vi "短信告警.vi"   [LabVIEW 2016]
uses:
  API/RND/example/Process var.vi
types:
  T1 = cluster{"水样参数输出":cluster{"mean":dbl, "变异系数":dbl, "随机数？":bool}, "零点参数输出":cluster{"mean":dbl, "变异系数":dbl, "随机数？":bool}, "跨度参数输出":cluster{"mean":dbl, "变异系数":dbl, "随机数？":bool}}
  T2 = cluster{"系统时间":timestamp, "工作状态":enum16{"空闲", "水样测试", "标样核查", "零点核查", "跨度核查", "空白测试", "平行样测试", "加标回收", "空白校准", "标样校准", "初始化（清洗）"}, "测量模式":enum16{"待机", "连续模式", "周期模式", "定点模式", "受控模式", "手动模式"}, "告警代码":u16, "故障代码":u16, "日志代码":u16, "软件版本":u16, "F0":sgl, "F1":sgl, "F2":sgl, "F3":sgl, "T":sgl, "H":sgl, "id":u16, "flowid":u16, "量程":u16, "总磷控温温度1":sgl, "营养盐控温温度2":sgl, "ADC":sgl}
  T3 = enum16{"空闲", "水样测试", "标样核查", "零点核查", "跨度核查", "空白测试", "平行样测试", "加标回收", "空白校准", "标样校准", "初始化（清洗）"}
  T4 = cluster{"参数":string, "报警内容":string, "报警分析":string}
  T5 = cluster{"系统时间":timestamp, "工作状态":u16, "测量模式":u16, "告警代码":u16, "故障代码":u16, "日志代码":u16, "软件版本":u16, "F0":sgl, "F1":sgl, "F2":sgl, "F3":sgl, "T":sgl, "H":sgl, "id":u16, "flowid":u16, "量程":u16}
  T6 = cluster{"ORP故障":bool, "温控器故障":bool, "加热故障":bool, "高锰酸钾报警":bool, "草酸钠报警":bool, "测量错误":bool, "校零错误":bool, "校标错误":bool, " 进水样超量程":bool, "排液阀故障":bool, "60分钟超时报警":bool, "进样无液体报警":bool}
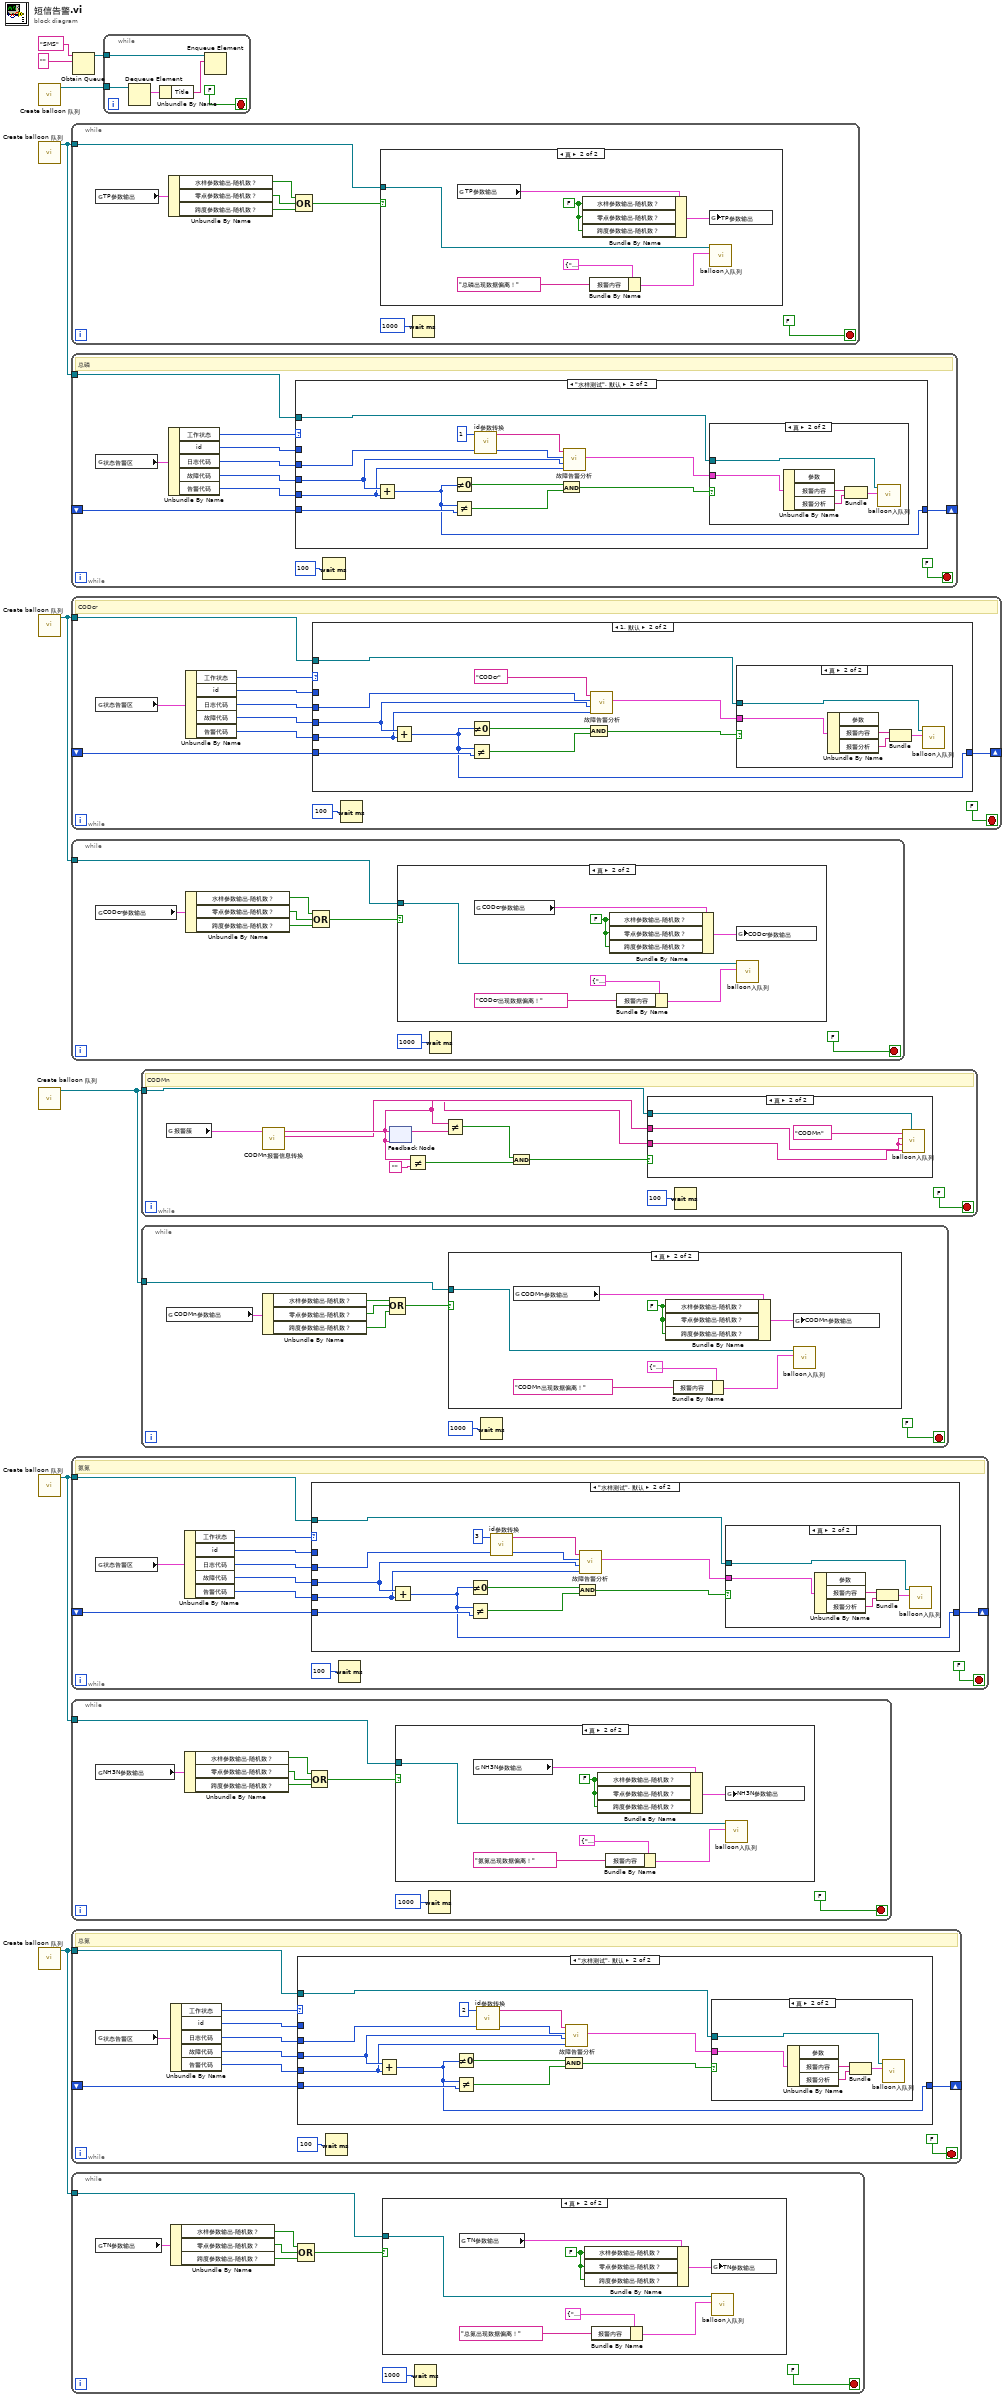
[diagram p0: block diagram]
diagram:
  n1 = call "Create balloon 队列.vi"() -> ("队列输出"=w9:refnum<queue>)  [unwired: 11 in]
  n2 = call "Create balloon 队列.vi"() -> ("队列输出"=w5:refnum<queue>)  [unwired: 11 in]
  n3 = call "Create balloon 队列.vi"() -> ("队列输出"=w4:refnum<queue>)  [unwired: 11 in]
  n4 = call "Create balloon 队列.vi"() -> ("队列输出"=w3:refnum<queue>)  [unwired: 11 in]
  n5 = call "Create balloon 队列.vi"() -> ("队列输出"=w2:refnum<queue>)  [unwired: 11 in]
  n6 = call "Create balloon 队列.vi"() -> ("队列输出"=w1:refnum<queue>)  [unwired: 11 in]
  n7 = while {
    tunnel: w5 -> [w10]
    stop <- FALSE stop-if-true
    n8 = global read "Process var.vi" "TP参数输出"() -> (w16:T1)
    n9 = Unbundle By Name(w16) -> ("水样参数输出.随机数？"=w15:bool, "零点参数输出.随机数？"=w14:bool, "跨度参数输出.随机数？"=w13:bool)
    n10 = Compound Arithmetic op=OR ("复合运算")(w15, w14, w13) -> (w12:bool)
    n11 = case shown="真" w12 {
      tunnel: w10 -> [_ w21]
      frame False {
      }
      frame True {
        w24 = FALSE ("水样参数输出.随机数？")
        n12 = global read "Process var.vi" "TP参数输出"() -> (w22:T1)
        n13 = Bundle By Name(cluster=w22, "水样参数输出.随机数？"=w24, "零点参数输出.随机数？"=w24, "跨度参数输出.随机数？"=w24) -> (w23:T1)
        n14 = Bundle By Name(cluster=cluster{"报警内容":string, "报警分析":string} {"报警内容"="", "报警分析"=""} ("报警内容"), "报警内容"="总磷出现数据偏离！") -> (w19:cluster{"报警内容":string, "报警分析":string})
        n15 = global write "Process var.vi" "TP参数输出"(w23) -> ()
        n16 = call "balloon入队列.vi"("报警内容"=w19, "队列"=w21) -> ()  [unwired: 9 in, 1 out]
      }
    }
    n17 = Wait (ms)(milliseconds to wait=u32 1000 ("等待时间（毫秒）")) -> ()  [unwired: 1 out]
  }
  n18 = while {
    tunnel: w5 -> [w31]
    shift-right: [w27] -> _
    shift-left: _ -> [w28]
    stop <- FALSE stop-if-true
    # "总磷"
    n19 = global read "VAR总磷总氮全局变量.vi" "状态告警区"() -> (w25:T2)
    n20 = Unbundle By Name(w25) -> ("工作状态"=w26:T3, "id"=w33:u16, "日志代码"=w32:u16, "故障代码"=w30:u16, "告警代码"=w29:u16)
    n21 = case shown="\"水样测试\", 默认" w26 {
      tunnel: w33 -> [_ _]
      tunnel: w32 -> [_ w48]
      tunnel: w31 -> [_ w45]
      tunnel: w30 -> [_ w44]
      tunnel: w29 -> [_ w43]
      tunnel: w28 -> [w36 w42]
      tunnel: [w36 w41] -> w27
      frame "空闲" {
      }
      frame "水样测试", Default {
        n22 = Add(x=w44, y=w43) -> (x+y=w41:u16)
        n23 = Not Equal To 0?(x=w41) -> (x != 0?=w40:bool)
        n24 = Not Equal?(x=w41, y=w42) -> (x != y?=w39:bool)
        n25 = call "id参数转换.vi"("id"=u16 1) -> ("table输出"=w46:string)  [unwired: 10 in]
        n26 = And(x=w40, y=w39) -> (x .and. y?=w38:bool)
        n27 = call "故障告警分析.vi"("告警代码"=w43, "故障代码"=w44, "运行步序"=w48, "参数"=w46) -> ("报警内容"=w47:T4)  [unwired: 6 in, 1 out]
        n28 = case shown="真" w38 {
          tunnel: w47 -> [_ w53]
          tunnel: w45 -> [_ w52]
          frame False {
          }
          frame True {
            n29 = Unbundle By Name(w53) -> ("报警内容"=w51:string, "报警分析"=w50:string)  [unwired: 1 out]
            n30 = Bundle("报警内容"=w51, "报警分析"=w50) -> (w49:cluster{"报警内容":string, "报警分析":string})  [unwired: 1 in]
            n31 = call "balloon入队列.vi"("报警内容"=w49, "队列"=w52) -> ()  [unwired: 9 in, 1 out]
          }
        }
      }
    }
    n32 = Wait (ms)(milliseconds to wait=u32 100) -> ()  [unwired: 1 out]
  }
  n33 = while {
    tunnel: w4 -> [w60]
    shift-right: [w56] -> _
    shift-left: _ -> [w57]
    stop <- FALSE stop-if-true
    # "CODcr"
    n34 = global read "CODcr全局变量.vi" "状态告警区"() -> (w54:T5)
    n35 = Unbundle By Name(w54) -> ("工作状态"=w55:u16, "id"=w62:u16, "日志代码"=w61:u16, "故障代码"=w59:u16, "告警代码"=w58:u16)
    n36 = case shown="1, 默认" w55 {
      tunnel: w62 -> [_ _]
      tunnel: w61 -> [_ w76]
      tunnel: w60 -> [_ w74]
      tunnel: w59 -> [_ w73]
      tunnel: w58 -> [_ w72]
      tunnel: w57 -> [w65 w71]
      tunnel: [w65 w70] -> w56
      frame 0 {
      }
      frame 1, Default {
        n37 = Add(x=w73, y=w72) -> (x+y=w70:u16)
        n38 = Not Equal To 0?(x=w70) -> (x != 0?=w69:bool)
        n39 = Not Equal?(x=w70, y=w71) -> (x != y?=w68:bool)
        n40 = And(x=w69, y=w68) -> (x .and. y?=w67:bool)
        n41 = call "故障告警分析.vi"("告警代码"=w72, "故障代码"=w73, "运行步序"=w76, "参数"="CODcr") -> ("报警内容"=w75:T4)  [unwired: 6 in, 1 out]
        n42 = case shown="真" w67 {
          tunnel: w75 -> [_ w81]
          tunnel: w74 -> [_ w80]
          frame False {
          }
          frame True {
            n43 = Unbundle By Name(w81) -> ("报警内容"=w79:string, "报警分析"=w78:string)  [unwired: 1 out]
            n44 = Bundle("报警内容"=w79, "报警分析"=w78) -> (w77:cluster{"报警内容":string, "报警分析":string})  [unwired: 1 in]
            n45 = call "balloon入队列.vi"("报警内容"=w77, "队列"=w80) -> ()  [unwired: 9 in, 1 out]
          }
        }
      }
    }
    n46 = Wait (ms)(milliseconds to wait=u32 100) -> ()  [unwired: 1 out]
  }
  n47 = while {
    tunnel: w4 -> [w82]
    stop <- FALSE stop-if-true
    n48 = global read "Process var.vi" "CODcr参数输出"() -> (w88:T1)
    n49 = Unbundle By Name(w88) -> ("水样参数输出.随机数？"=w87:bool, "零点参数输出.随机数？"=w86:bool, "跨度参数输出.随机数？"=w85:bool)
    n50 = Compound Arithmetic op=OR ("复合运算")(w87, w86, w85) -> (w84:bool)
    n51 = case shown="真" w84 {
      tunnel: w82 -> [_ w93]
      frame False {
      }
      frame True {
        w96 = FALSE ("水样参数输出.随机数？")
        n52 = global read "Process var.vi" "CODcr参数输出"() -> (w94:T1)
        n53 = Bundle By Name(cluster=w94, "水样参数输出.随机数？"=w96, "零点参数输出.随机数？"=w96, "跨度参数输出.随机数？"=w96) -> (w95:T1)
        n54 = Bundle By Name(cluster=cluster{"报警内容":string, "报警分析":string} {"报警内容"="", "报警分析"=""} ("报警内容"), "报警内容"="CODcr出现数据偏离！") -> (w91:cluster{"报警内容":string, "报警分析":string})
        n55 = global write "Process var.vi" "CODcr参数输出"(w95) -> ()
        n56 = call "balloon入队列.vi"("报警内容"=w91, "队列"=w93) -> ()  [unwired: 9 in, 1 out]
      }
    }
    n57 = Wait (ms)(milliseconds to wait=u32 1000 ("等待时间（毫秒）")) -> ()  [unwired: 1 out]
  }
  n58 = while {
    tunnel: w2 -> [w103]
    shift-right: [w99] -> _
    shift-left: _ -> [w100]
    stop <- FALSE stop-if-true
    # "氨氮"
    n59 = global read "VAR氨氮全局变量.vi" "状态告警区"() -> (w97:T2)
    n60 = Unbundle By Name(w97) -> ("工作状态"=w98:T3, "id"=w105:u16, "日志代码"=w104:u16, "故障代码"=w102:u16, "告警代码"=w101:u16)
    n61 = case shown="\"水样测试\", 默认" w98 {
      tunnel: w105 -> [_ _]
      tunnel: w104 -> [_ w120]
      tunnel: w103 -> [_ w117]
      tunnel: w102 -> [_ w116]
      tunnel: w101 -> [_ w115]
      tunnel: w100 -> [w108 w114]
      tunnel: [w108 w113] -> w99
      frame "空闲" {
      }
      frame "水样测试", Default {
        n62 = Add(x=w116, y=w115) -> (x+y=w113:u16)
        n63 = Not Equal To 0?(x=w113) -> (x != 0?=w112:bool)
        n64 = Not Equal?(x=w113, y=w114) -> (x != y?=w111:bool)
        n65 = call "id参数转换.vi"("id"=u16 3) -> ("table输出"=w118:string)  [unwired: 10 in]
        n66 = And(x=w112, y=w111) -> (x .and. y?=w110:bool)
        n67 = call "故障告警分析.vi"("告警代码"=w115, "故障代码"=w116, "运行步序"=w120, "参数"=w118) -> ("报警内容"=w119:T4)  [unwired: 6 in, 1 out]
        n68 = case shown="真" w110 {
          tunnel: w119 -> [_ w125]
          tunnel: w117 -> [_ w124]
          frame False {
          }
          frame True {
            n69 = Unbundle By Name(w125) -> ("报警内容"=w123:string, "报警分析"=w122:string)  [unwired: 1 out]
            n70 = Bundle("报警内容"=w123, "报警分析"=w122) -> (w121:cluster{"报警内容":string, "报警分析":string})  [unwired: 1 in]
            n71 = call "balloon入队列.vi"("报警内容"=w121, "队列"=w124) -> ()  [unwired: 9 in, 1 out]
          }
        }
      }
    }
    n72 = Wait (ms)(milliseconds to wait=u32 100) -> ()  [unwired: 1 out]
  }
  n73 = while {
    tunnel: w2 -> [w126]
    stop <- FALSE stop-if-true
    n74 = global read "Process var.vi" "NH3N参数输出"() -> (w132:T1)
    n75 = Unbundle By Name(w132) -> ("水样参数输出.随机数？"=w131:bool, "零点参数输出.随机数？"=w130:bool, "跨度参数输出.随机数？"=w129:bool)
    n76 = Compound Arithmetic op=OR ("复合运算")(w131, w130, w129) -> (w128:bool)
    n77 = case shown="真" w128 {
      tunnel: w126 -> [_ w137]
      frame False {
      }
      frame True {
        w140 = FALSE ("水样参数输出.随机数？")
        n78 = global read "Process var.vi" "NH3N参数输出"() -> (w138:T1)
        n79 = Bundle By Name(cluster=w138, "水样参数输出.随机数？"=w140, "零点参数输出.随机数？"=w140, "跨度参数输出.随机数？"=w140) -> (w139:T1)
        n80 = Bundle By Name(cluster=cluster{"报警内容":string, "报警分析":string} {"报警内容"="", "报警分析"=""} ("报警内容"), "报警内容"="氨氮出现数据偏离！") -> (w135:cluster{"报警内容":string, "报警分析":string})
        n81 = global write "Process var.vi" "NH3N参数输出"(w139) -> ()
        n82 = call "balloon入队列.vi"("报警内容"=w135, "队列"=w137) -> ()  [unwired: 9 in, 1 out]
      }
    }
    n83 = Wait (ms)(milliseconds to wait=u32 1000 ("等待时间（毫秒）")) -> ()  [unwired: 1 out]
  }
  n84 = while {
    tunnel: w1 -> [w147]
    shift-right: [w143] -> _
    shift-left: _ -> [w144]
    stop <- FALSE stop-if-true
    # "总氮"
    n85 = global read "VAR总磷总氮全局变量.vi" "状态告警区"() -> (w141:T2)
    n86 = Unbundle By Name(w141) -> ("工作状态"=w142:T3, "id"=w149:u16, "日志代码"=w148:u16, "故障代码"=w146:u16, "告警代码"=w145:u16)
    n87 = case shown="\"水样测试\", 默认" w142 {
      tunnel: w149 -> [_ _]
      tunnel: w148 -> [_ w164]
      tunnel: w147 -> [_ w161]
      tunnel: w146 -> [_ w160]
      tunnel: w145 -> [_ w159]
      tunnel: w144 -> [w152 w158]
      tunnel: [w152 w157] -> w143
      frame "空闲" {
      }
      frame "水样测试", Default {
        n88 = Add(x=w160, y=w159) -> (x+y=w157:u16)
        n89 = Not Equal To 0?(x=w157) -> (x != 0?=w156:bool)
        n90 = Not Equal?(x=w157, y=w158) -> (x != y?=w155:bool)
        n91 = call "id参数转换.vi"("id"=u16 2) -> ("table输出"=w162:string)  [unwired: 10 in]
        n92 = And(x=w156, y=w155) -> (x .and. y?=w154:bool)
        n93 = call "故障告警分析.vi"("告警代码"=w159, "故障代码"=w160, "运行步序"=w164, "参数"=w162) -> ("报警内容"=w163:T4)  [unwired: 6 in, 1 out]
        n94 = case shown="真" w154 {
          tunnel: w163 -> [_ w169]
          tunnel: w161 -> [_ w168]
          frame False {
          }
          frame True {
            n95 = Unbundle By Name(w169) -> ("报警内容"=w167:string, "报警分析"=w166:string)  [unwired: 1 out]
            n96 = Bundle("报警内容"=w167, "报警分析"=w166) -> (w165:cluster{"报警内容":string, "报警分析":string})  [unwired: 1 in]
            n97 = call "balloon入队列.vi"("报警内容"=w165, "队列"=w168) -> ()  [unwired: 9 in, 1 out]
          }
        }
      }
    }
    n98 = Wait (ms)(milliseconds to wait=u32 100) -> ()  [unwired: 1 out]
  }
  n99 = while {
    tunnel: w1 -> [w170]
    stop <- FALSE stop-if-true
    n100 = global read "Process var.vi" "TN参数输出"() -> (w176:T1)
    n101 = Unbundle By Name(w176) -> ("水样参数输出.随机数？"=w175:bool, "零点参数输出.随机数？"=w174:bool, "跨度参数输出.随机数？"=w173:bool)
    n102 = Compound Arithmetic op=OR ("复合运算")(w175, w174, w173) -> (w172:bool)
    n103 = case shown="真" w172 {
      tunnel: w170 -> [_ w181]
      frame False {
      }
      frame True {
        w184 = FALSE ("水样参数输出.随机数？")
        n104 = global read "Process var.vi" "TN参数输出"() -> (w182:T1)
        n105 = Bundle By Name(cluster=w182, "水样参数输出.随机数？"=w184, "零点参数输出.随机数？"=w184, "跨度参数输出.随机数？"=w184) -> (w183:T1)
        n106 = Bundle By Name(cluster=cluster{"报警内容":string, "报警分析":string} {"报警内容"="", "报警分析"=""} ("报警内容"), "报警内容"="总氮出现数据偏离！") -> (w179:cluster{"报警内容":string, "报警分析":string})
        n107 = global write "Process var.vi" "TN参数输出"(w183) -> ()
        n108 = call "balloon入队列.vi"("报警内容"=w179, "队列"=w181) -> ()  [unwired: 9 in, 1 out]
      }
    }
    n109 = Wait (ms)(milliseconds to wait=u32 1000 ("等待时间（毫秒）")) -> ()  [unwired: 1 out]
  }
  n110 = Obtain Queue(name (unnamed)="SMS" ("名称（未命名）"), element data type="" ("名称（未命名）")) -> (queue out=w6:refnum<queue>)  [unwired: 3 in, 2 out]
  n111 = while {
    tunnel: w9 -> [w188]
    tunnel: w6 -> [w187]
    stop <- FALSE stop-if-true
    n112 = Dequeue Element(queue=w188) -> (element=w186:cluster{"Title":string, "Body":string})  [unwired: 2 in, 3 out]
    n113 = Unbundle By Name(w186) -> ("Title"=w185:string)
    n114 = Enqueue Element(queue=w187, element=w185) -> ()  [unwired: 2 in, 3 out]
  }
  n115 = while {
    tunnel: w3 -> [w191]
    stop <- FALSE stop-if-true
    # "CODMn"
    n116 = global read "COD内部交互全局.vi" "报警簇"() -> (w194:T6)
    n117 = call "CODMn报警信息转换.vi"("报警簇"=w194) -> ("CODMN报警信息备注"=w193:string, "CODMN报警信息"=w195:string)  [unwired: 9 in]
    n118 = feedback #1(w195) -> (w196:string)
    n119 = feedback-in #1(w195) -> ()
    n120 = Not Equal?(x=w195, y="") -> (x != y?=w200:bool)
    n121 = Not Equal?(x=w195, y=w196) -> (x != y?=w197:bool)
    n122 = And(x=w197, y=w200) -> (x .and. y?=w198:bool)
    n123 = case shown="真" w198 {
      tunnel: w195 -> [_ w202]
      tunnel: w193 -> [_ w203]
      tunnel: w191 -> [_ w204]
      frame False {
      }
      frame True {
        n124 = call "balloon入队列.vi"("队列"=w204, "故障详情"=w203, "告警信息"=w202, "故障信息"=w202, "参数名称"="CODMn") -> ()  [unwired: 6 in, 1 out]
      }
    }
    n125 = Wait (ms)(milliseconds to wait=u32 100) -> ()  [unwired: 1 out]
  }
  n126 = while {
    tunnel: w3 -> [w205]
    stop <- FALSE stop-if-true
    n127 = global read "Process var.vi" "CODMn参数输出"() -> (w211:T1)
    n128 = Unbundle By Name(w211) -> ("水样参数输出.随机数？"=w210:bool, "零点参数输出.随机数？"=w209:bool, "跨度参数输出.随机数？"=w208:bool)
    n129 = Compound Arithmetic op=OR ("复合运算")(w210, w209, w208) -> (w207:bool)
    n130 = case shown="真" w207 {
      tunnel: w205 -> [_ w216]
      frame False {
      }
      frame True {
        w219 = FALSE ("水样参数输出.随机数？")
        n131 = global read "Process var.vi" "CODMn参数输出"() -> (w217:T1)
        n132 = Bundle By Name(cluster=w217, "水样参数输出.随机数？"=w219, "零点参数输出.随机数？"=w219, "跨度参数输出.随机数？"=w219) -> (w218:T1)
        n133 = Bundle By Name(cluster=cluster{"报警内容":string, "报警分析":string} {"报警内容"="", "报警分析"=""} ("报警内容"), "报警内容"="CODMn出现数据偏离！") -> (w214:cluster{"报警内容":string, "报警分析":string})
        n134 = global write "Process var.vi" "CODMn参数输出"(w218) -> ()
        n135 = call "balloon入队列.vi"("报警内容"=w214, "队列"=w216) -> ()  [unwired: 9 in, 1 out]
      }
    }
    n136 = Wait (ms)(milliseconds to wait=u32 1000 ("等待时间（毫秒）")) -> ()  [unwired: 1 out]
  }
